vi "arduino_only.vi"() -> ()   [LabVIEW 2012]
panel:
  in  "Tab Control":T1(tab)
  in  "VISA resource name":refnum<visa-resource-name>="COM3"
  in  "Slow Control On":bool
  in  "Write Enable":bool
  in  "File Path":path=path "D:/Users/reuterc/Desktop"
  out "directory exists - please wait":u8(slide)
  out "directory ok":bool
  in  "General Cluster":cluster{"Location":i16} {"Location" items=["Purdue", "NIKHEF", "Zurich", "???"]}
  in  "IP Address of NIST Time Server":string(combo)
  in  "HV Cluster":T2={"HV Power On/Off"=[], "Set Voltage"=[], "HV Tolerance (%)"=1.0}
  out "Slow Cluster":T3
  out "data":dbl[](array[numeric])
  in  "XOFF Character":u8=19 format="%.0x"
  in  "XON Character":u8=17 format="%.0x"
  in  "Arduino read rate (Hz)":dbl=1.0
  out "Arduino \nread failed":bool
  out "UTC format":bool=TRUE
  out "read buffer":string
  out "Temperature":dbl(graph)
  out "Pressure":dbl(graph)
  out "total magnetic field":dbl(graph)
  out "magnetic field z coordinate":dbl(graph)
  out "magnetic field y coordinate":dbl(graph)
  out "magnetic field x coordinate":dbl(graph)
  out "humidity":dbl(graph)
  out "Slow XML":string
  out "NIST Time":u64
  out "Slow time":u64
  in  "Minutes to wait":u32=5 min=3
  out "NIST Time Failed to Read":bool
  out "created path":path
  out "File name":string
  out "Stopped":bool
  in  "stop 2":bool
  in  "stop":bool
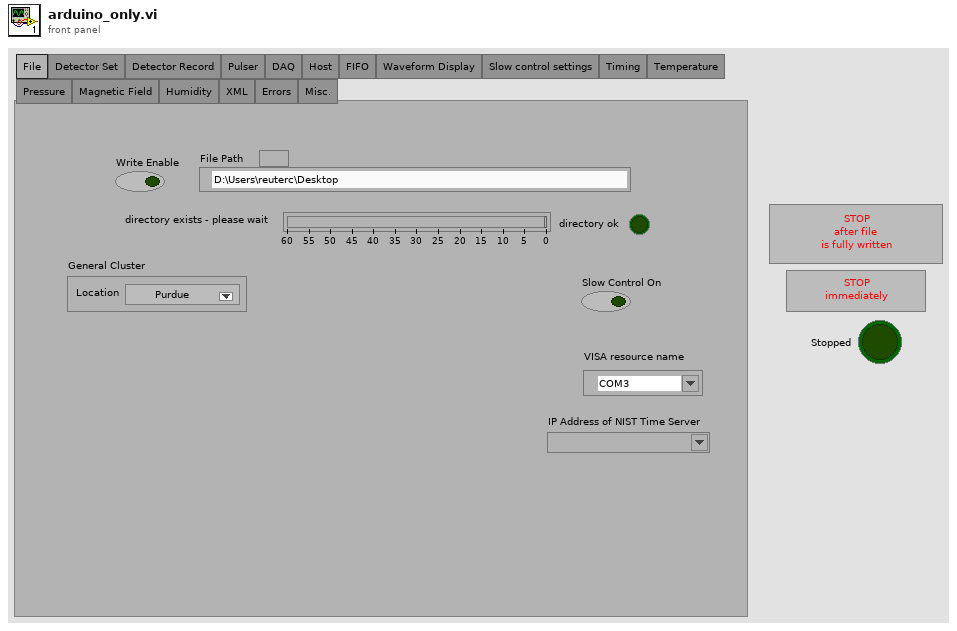
[diagram p1: front panel]
types:
  T1 = enum32{"File", "Detector Set", "Detector Record", "Pulser", "DAQ", "Host", "FIFO", "Waveform Display", "Slow control settings", "Timing", "Temperature", "Pressure", "Magnetic Field", "Humidity", "XML", "Errors", "Misc."}
  T2 = cluster{"HV Power On/Off":bool[], "Set Voltage":string[], "HV Tolerance (%)":dbl}
  T3 = cluster{"Arduino Parameters":dbl, "Total Number of Slow Parameters":i32, "UTC format?":bool, "Sensor Upper bounds":i32[], "Sensor Lower bounds":i32[], "Descriptions":string[], "datanames":string[]}
  T4 = enum16{"open", "replace", "create", "open or create", "replace or create", "replace or create with confirmation"}
  T5 = enum16{"big-endian, network order", "native, host order", "little-endian"}
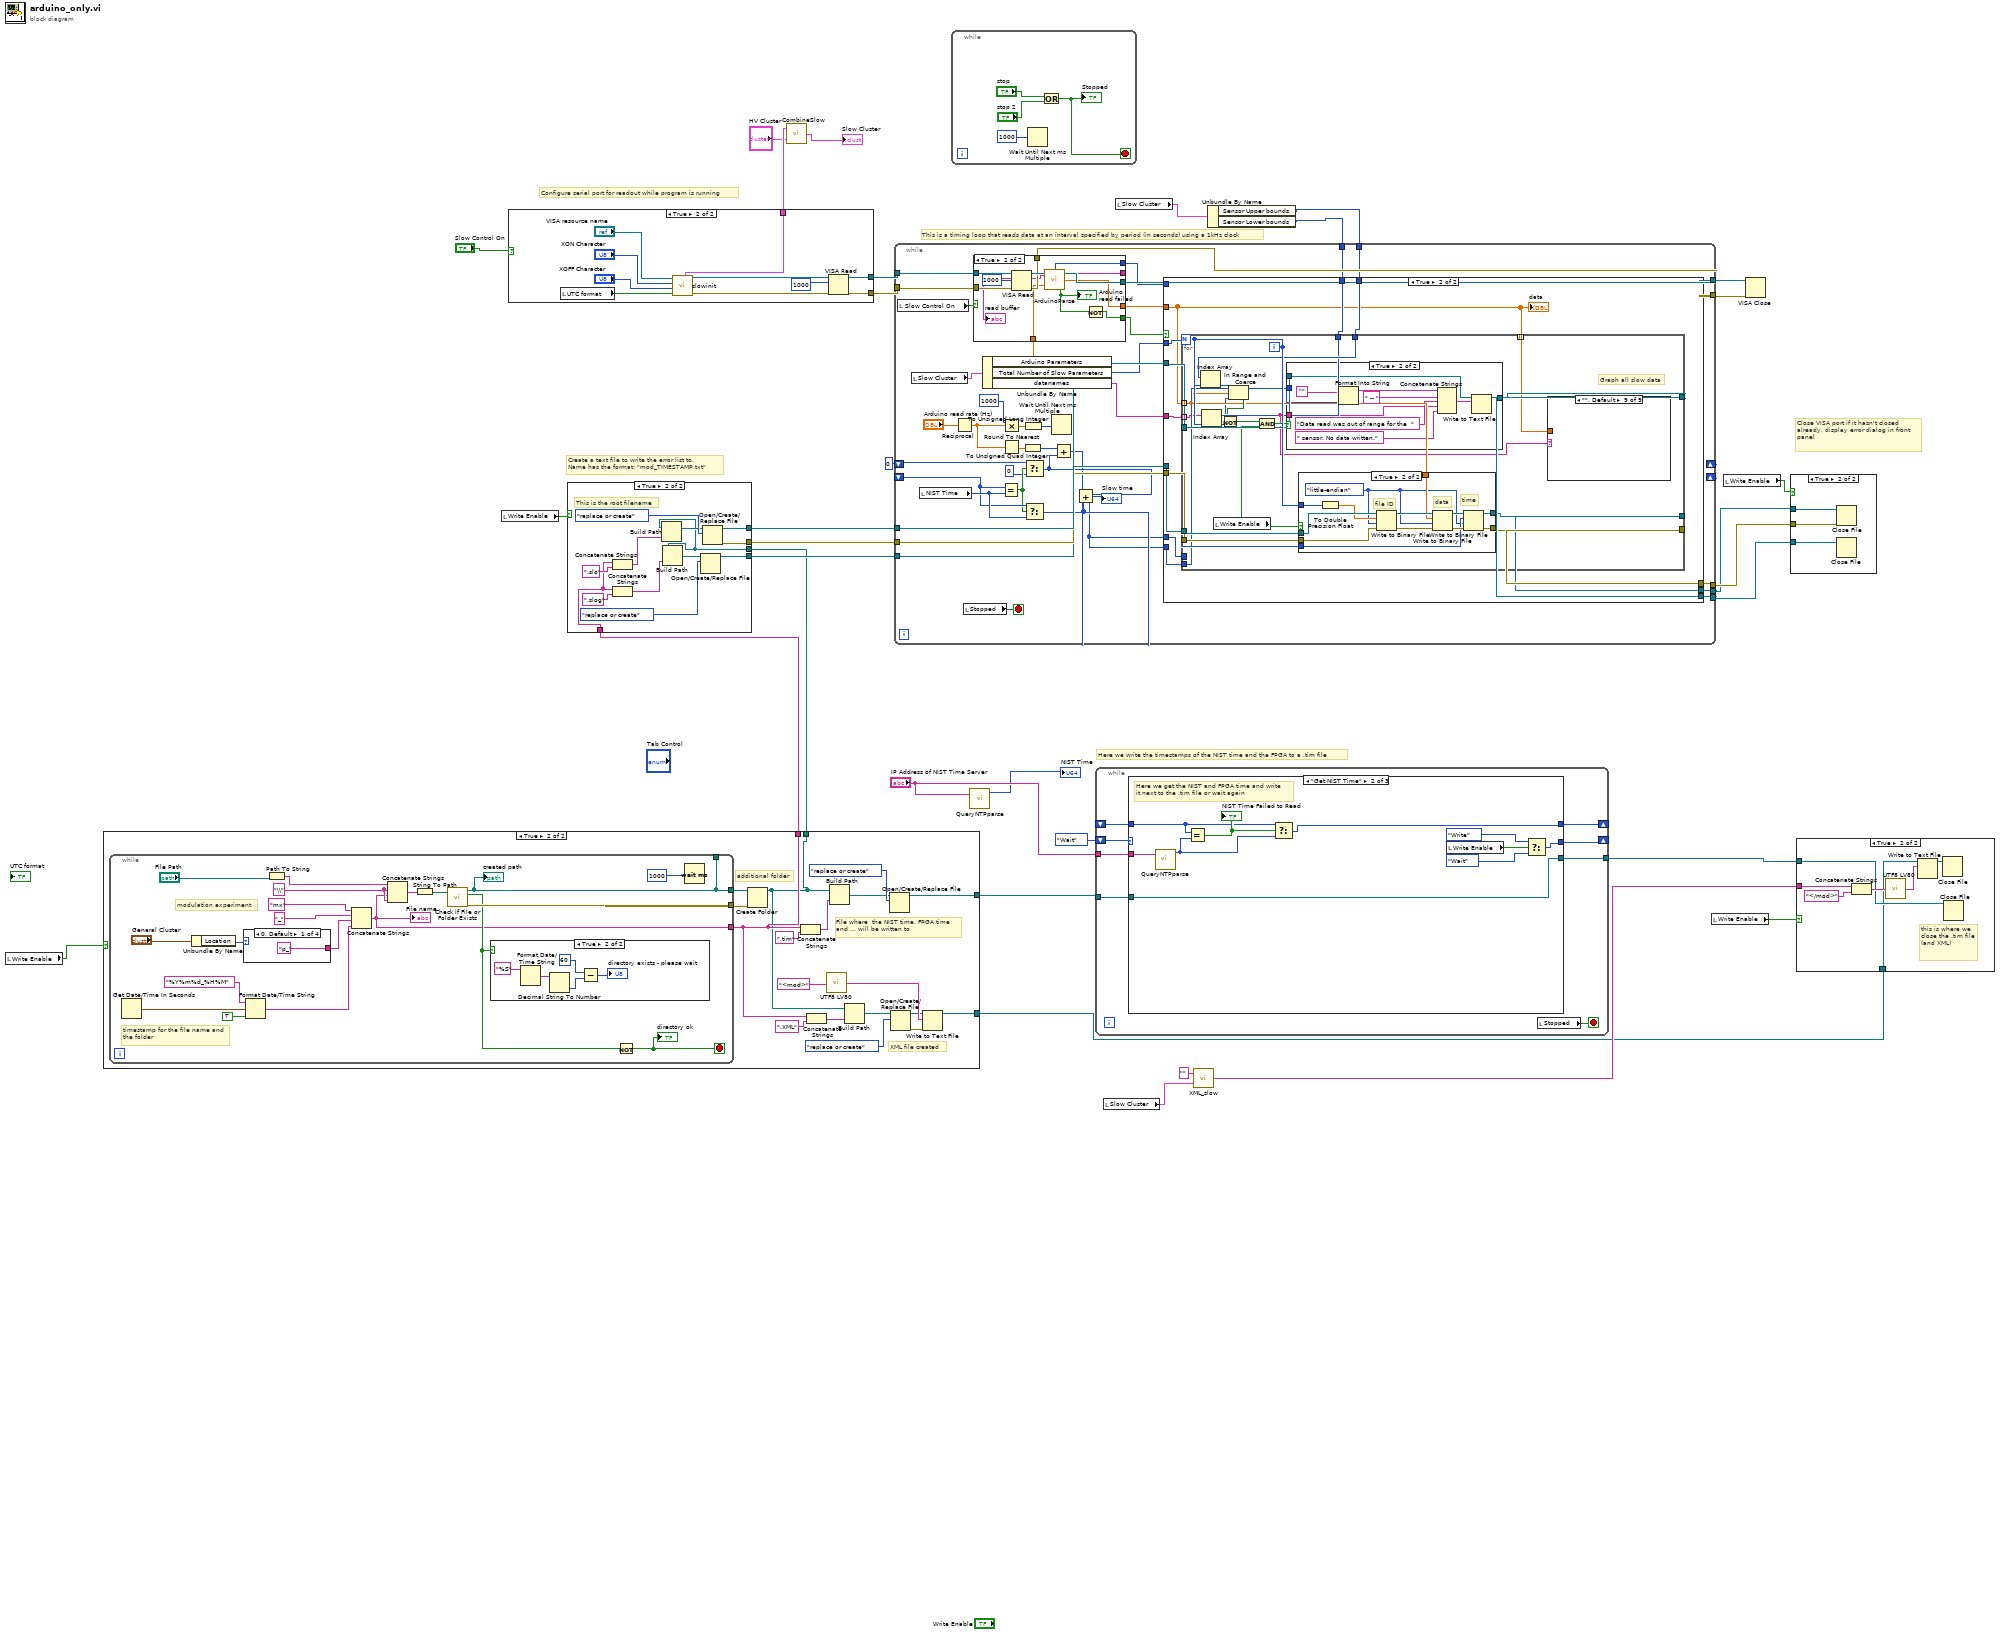
[diagram p0: block diagram]
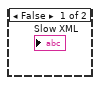
[diagram p3: hidden frame]
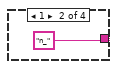
[diagram p4: hidden frame]
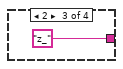
[diagram p5: hidden frame]
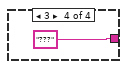
[diagram p6: hidden frame]
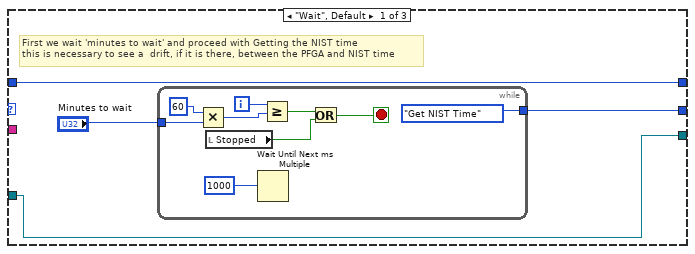
[diagram p8: hidden frame]
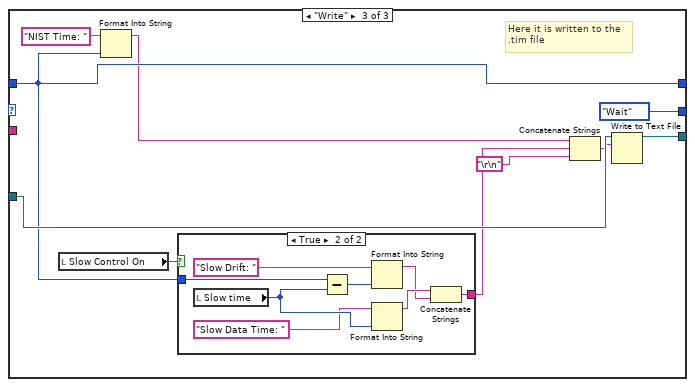
[diagram p9: hidden frame]
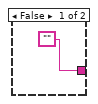
[diagram p10: hidden frame]
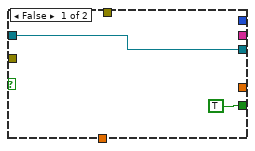
[diagram p12: hidden frame]
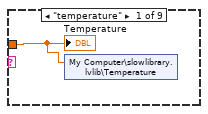
[diagram p14: hidden frame]
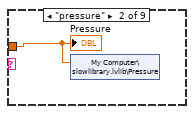
[diagram p15: hidden frame]
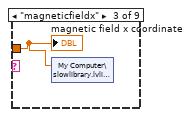
[diagram p16: hidden frame]
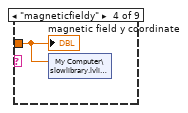
[diagram p17: hidden frame]
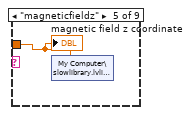
[diagram p18: hidden frame]
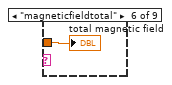
[diagram p19: hidden frame]
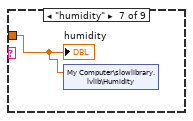
[diagram p20: hidden frame]
diagram:
  # "Here we write the timestamps of the NIST time and the FPGA to a .tim file"
  # "Create a text file to write the error list to.  \nName has the format: \"mod_TIMESTAMP.txt\""
  # "This is a timing loop that reads data at an interval specified by period (in seconds) using a 1kHz clock"
  # "Configure serial port for readout while program is running"
  # "Close VISA port if it hasn't closed already, display error dialog in front panel"
  n1 = local read "Write Enable"() -> (w4:bool)
  n2 = case shown="True" w4 {
    tunnel: [_ w38] -> w11
    tunnel: [_ w37] -> w5
    tunnel: [_ w36] -> w3
    tunnel: [_ w34] -> w1
    frame False {
    }
    frame True {
      # "XML file created"
      # "File where  the NIST time, FPGA time\nand ... will be written to"
      # "additional folder"
      n3 = while {
        tunnel: [w64] -> w47
        tunnel: [w56] -> w48
        tunnel: [w56] -> _
        tunnel: [w55] -> w36
        stop <- w61 stop-if-true
        w57 = "\\" ("string")
        # "modulation experiment"
        # "timestamp for the file name and the folder"
        n4 = Get Date/Time In Seconds() -> (seconds since 1Jan1904=w68:timestamp)
        n5 = Unbundle By Name("General Cluster") -> ("Location"=w53:i16)
        n6 = case shown="0, Default" w53 {
          tunnel: ["p_" ("string") "n_" ("string") "z_" ("string") "???"] -> w54
          frame 0, Default {
          }
          frame 1 {
          }
          frame 2 {
          }
          frame 3 {
          }
        }
        n7 = Format Date/Time String(time format string (%c)="%Y%m%d_%H%M", seconds (now)=w68, UTC format=TRUE) -> (date/time string=w58:string)
        n8 = Path To String(path="File Path") -> (string=w70:string)
        n9 = Concatenate Strings("mx" ("string"), "_" ("string"), w54, w58) -> (w55:string)
        "File name" <- w55
        n10 = Concatenate Strings(w70, w57, w55, w57) -> (w71:string)
        n11 = String To Path(string=w71) -> (path=w65:path)
        n12 = call <vilib>:"Check if File or Folder Exists.vi"("path"=w65) -> ("error out"=w64:errorcluster, "file or folder exists?"=w63:bool, "dup path"=w56:path)  [unwired: 8 in]
        "created path" <- w56
        n13 = case shown="True" w63 {
          frame False {
          }
          frame True {
            n14 = Format Date/Time String(time format string (%c)="%S") -> (date/time string=w79:string)  [unwired: 2 in]
            n15 = Decimal String To Number(string=w79) -> (number=w77:i32)  [unwired: 2 in, 1 out]
            n16 = Subtract(x=60, y=w77) -> (x-y=→"directory exists - please wait":i32)
          }
        }
        n17 = Not(x=w63) -> (.not. x?=w61:bool)
        "directory ok" <- w61
        n18 = Wait (ms)(milliseconds to wait=1000) -> ()  [unwired: 1 out]
      }
      n19 = Create Folder(path (use dialog)=w48, error in=w47) -> (created path=w34:path)  [unwired: 1 in, 2 out]
      n20 = Concatenate Strings(w36, ".tim" ("string")) -> (w49:string)
      n21 = Concatenate Strings(w36, ".XML" ("substring (\"\")")) -> (w43:string)
      n22 = call "UTF8 LV80.vi"("text"="<mod>") -> ("utf-8 text out"=w46:string)
      n23 = Build Path(base path=w34, name or relative path=w49) -> (appended path=w35:path)
      n24 = Build Path(base path=w34, name or relative path=w43) -> (appended path=w42:path)
      n25 = Open/Create/Replace File(file path (use dialog)=w35, operation (0:open)=T4."replace or create") -> (refnum out=w38:refnum<file>)  [unwired: 4 in, 2 out]
      n26 = Open/Create/Replace File(file path (use dialog)=w42, operation (0:open)=T4."replace or create") -> (refnum out=w45:refnum<file>, error out=w44:errorcluster)  [unwired: 4 in, 1 out]
      n27 = Write to Text File(file (use dialog)=w45, text=w46, error in=w44) -> (refnum out=w37:refnum<file>)  [unwired: 1 in, 2 out]
    }
  }
  n28 = local read "Write Enable"() -> (w32:bool)
  n29 = case shown="True" "Slow Control On" {
    tunnel: [_ w90] -> w24
    tunnel: [_ w89] -> w23
    tunnel: [_ w81] -> w16
    frame False {
    }
    frame True {
      n30 = local read "UTC format"() -> (w84:bool)
      n31 = call "slowinit.vi"("UTC format"=w84, "XOFF Character"="XOFF Character", "XON Character"="XON Character", "VISA resource name"="VISA resource name") -> ("error IO"=w82:errorcluster, "VISA resource name out"=w83:refnum<visa-resource-name>, "Slow Cluster"=w81:T3)  [unwired: 5 in]
      n32 = VISA Read(VISA resource name=w83, byte count=u32 1000, error in (no error)=w82) -> (VISA resource name out=w90:refnum<visa-resource-name>, error out=w89:errorcluster)  [unwired: 2 out]
    }
  }
  n33 = case shown="True" w32 {
    tunnel: [_ w101] -> w29
    tunnel: [_ w98] -> w27
    tunnel: [_ w93] -> w22
    tunnel: w3 -> [_ w92]
    tunnel: w1 -> [_ w91]
    frame False {
    }
    frame True {
      # "This is the root filename"
      n34 = Concatenate Strings(w92, ".slo") -> (w99:string)
      n35 = Concatenate Strings(w92, ".slog") -> (w94:string)
      n36 = Build Path(base path=w91, name or relative path=w99) -> (appended path=w100:path)
      n37 = Build Path(base path=w91, name or relative path=w94) -> (appended path=w95:path)
      n38 = Open/Create/Replace File(file path (use dialog)=w95, operation (0:open)=T4."replace or create") -> (refnum out=w93:refnum<file>)  [unwired: 4 in, 2 out]
      n39 = Open/Create/Replace File(file path (use dialog)=w100, operation (0:open)=T4."replace or create") -> (refnum out=w101:refnum<file>, error out=w98:errorcluster)  [unwired: 4 in, 1 out]
    }
  }
  n40 = call "CombineSlow.vi"("HV Cluster"="HV Cluster", "Slow Cluster"=w16) -> ("Slow Cluster 2"=→"Slow Cluster":T3)
  n41 = while {
    stop <- w104 stop-if-true
    n42 = Wait Until Next ms Multiple(millisecond multiple=u32 1000 ("y")) -> ()  [unwired: 1 out]
    n43 = Or(x="stop", y="stop 2") -> (x .or. y?=w104:bool)
    "Stopped" <- w104
  }
  n44 = call "QueryNTPparse.vi"("IP Address of NIST Server"="IP Address of NIST Time Server") -> ("NTP Time"=→"NIST Time":u64)  [unwired: 1 in, 2 out]
  n45 = while {
    shift-right: [w114] -> _
    shift-left: enum16{"Wait", "Get NIST Time", "Write"}."Wait" -> [w115]
    shift-right: [w113] -> _
    shift-left: _ -> [w112]
    tunnel: w11 -> [w111]
    tunnel: [w110] -> w9
    tunnel: "IP Address of NIST Time Server" -> [w109]
    stop <- w108 stop-if-true
    n46 = case shown="\"Get NIST Time\"" w115 {
      tunnel: [w119 w130 enum16{"Wait", "Get NIST Time", "Write"}."Wait"] -> w114
      tunnel: [w118 w138 w143] -> w113
      tunnel: w112 -> [w118 w135 w143]
      tunnel: w111 -> [w117 w134 w147]
      tunnel: [w117 w134 w146] -> w110
      tunnel: w109 -> [_ w129 _]
      frame "Wait", Default {
        # "First we wait 'minutes to wait' and proceed with Getting the NIST time\nthis is necessary to see a  drift, if it is there, between the PFGA and NIST time"
        n47 = while {
          tunnel: [enum16{"Wait", "Get NIST Time", "Write"}."Get NIST Time"] -> w119
          tunnel: "Minutes to wait" -> [w122]
          i -> [w124]
          stop <- w125 stop-if-true
          n48 = Multiply(x=60, y=w122) -> (x*y=w121:u32)
          n49 = local read "Stopped"() -> (w120:bool)
          n50 = Wait Until Next ms Multiple(millisecond multiple=u32 1000 ("y")) -> ()  [unwired: 1 out]
          n51 = Greater Or Equal?(x=w124, y=w121) -> (x >= y?=w126:bool)
          n52 = Or(x=w126, y=w120) -> (x .or. y?=w125:bool)
        }
      }
      frame "Get NIST Time" {
        # "Here we get the NIST and FPGA time and write\nit next to the .tim file or wait again"
        n53 = call "QueryNTPparse.vi"("IP Address of NIST Server"=w129) -> ("NTP Time"=w137:u64)  [unwired: 1 in, 2 out]
        n54 = Equal?(x=w135, y=w137) -> (x = y?=w136:bool)
        "NIST Time Failed to Read" <- w136
        n55 = Select(t=w135, s=w136, f=w137) -> (s? t:f=w138:u64)
        n56 = local read "Write Enable"() -> (w133:bool)
        n57 = Select(t=enum16{"Wait", "Get NIST Time", "Write"}."Write", s=w133, f=enum16{"Wait", "Get NIST Time", "Write"}."Wait") -> (s? t:f=w130:enum16{"Wait", "Get NIST Time", "Write"})
      }
      frame "Write" {
        # "Here it is written to the \n.tim file"
        n58 = local read "Slow Control On"() -> (w140:bool)
        n59 = Format Into String(initial string="NIST Time: ", w143) -> (resulting string=w139:string)  [unwired: 2 in, 1 out]
        n60 = case shown="True" w140 {
          tunnel: w143 -> [_ w154]
          tunnel: ["" w150] -> w142
          frame False {
          }
          frame True {
            n61 = local read "Slow time"() -> (w157:u64)
            n62 = Subtract(x=w154, y=w157) -> (x-y=w153:u64)
            n63 = Format Into String(initial string="Slow Drift: ", w153) -> (resulting string=w151:string)  [unwired: 2 in, 1 out]
            n64 = Format Into String(initial string="Slow Data Time: ", w157) -> (resulting string=w152:string)  [unwired: 2 in, 1 out]
            n65 = Concatenate Strings(w152, w151) -> (w150:string)
          }
        }
        n66 = Concatenate Strings(w139, w142, "\r\n") -> (w145:string)
        n67 = Write to Text File(file (use dialog)=w147, text=w145) -> (refnum out=w146:refnum<file>)  [unwired: 2 in, 2 out]
      }
    }
    n68 = local read "Stopped"() -> (w108:bool)
  }
  n69 = local read "Slow Cluster"() -> (w7:T3)
  n70 = local read "Slow Cluster"() -> (w20:T3)
  n71 = call "XML_slow.vi"("Slow Cluster"=w7, "Input String"="") -> ("Output String"=w6:string)
  n72 = Unbundle By Name(w20) -> ("Sensor Upper bounds"=w19:i32[], "Sensor Lower bounds"=w18:i32[])
  n73 = while {
    tunnel: w24 -> [w194]
    tunnel: w23 -> [w193]
    tunnel: [w192] -> w31
    tunnel: [w191] -> w30
    shift-right: [w184] -> _
    shift-left: _ -> [w188]
    shift-right: [w173] -> _
    shift-left: 0 -> [w186]
    tunnel: w27 -> [w182]
    tunnel: [w181] -> w26
    tunnel: w29 -> [w190]
    tunnel: [w180] -> w25
    tunnel: w22 -> [w179]
    tunnel: [w177] -> w21
    tunnel: w19 -> [w165]
    tunnel: w18 -> [w164]
    stop <- w183 stop-if-true
    n74 = local read "Slow Control On"() -> (w161:bool)
    n75 = local read "Slow Cluster"() -> (w167:T3)
    n76 = local read "NIST Time"() -> (w189:u64)
    n77 = Reciprocal(x="Arduino read rate (Hz)") -> (1/x=w170:dbl)
    n78 = local read "Stopped"() -> (w183:bool)
    n79 = Unbundle By Name(w167) -> ("Arduino Parameters"=w162:dbl, "Total Number of Slow Parameters"=w163:i32, "datanames"=w159:string[])
    n80 = case shown="True" w161 {
      tunnel: w194 -> [w195 w207]
      tunnel: w193 -> [_ w206]
      tunnel: [w195 w205] -> w192
      tunnel: [_ w204] -> w191
      tunnel: [_ w202] -> w166
      tunnel: [_ w201] -> _
      tunnel: [TRUE w197] -> w160
      tunnel: [_ w199] -> w158
      tunnel: w162 -> [_ w198]
      frame False {
      }
      frame True {
        n81 = VISA Read(VISA resource name=w207, byte count=u32 1000, error in (no error)=w206) -> (VISA resource name out=w205:refnum<visa-resource-name>, read buffer=w203:string, error out=w204:errorcluster)  [unwired: 1 out]
        "read buffer" <- w203
        n82 = call "ArduinoParse.vi"("read buffer"=w203, "Expected Arduino Parameters"=w198) -> ("Number Arduino Parameters"=w202:i32, "Arduino Data Names"=w201:string[], "Arduino Data"=w199:dbl[], "Arduino Read Failed?"=w200:bool)
        "Arduino \nread failed" <- w200
        n83 = Not(x=w200) -> (.not. x?=w197:bool)
      }
    }
    n84 = Equal?(x=w188, y=w189) -> (x = y?=w187:bool)
    n85 = Multiply(x=u32 1000 ("millisecond multiple"), y=w170) -> (x*y=w172:dbl)
    n86 = Round To Nearest(number=w170) -> (nearest integer value=w169:dbl)
    n87 = To Unsigned Quad Integer(1:w169) -> (0:w168:u64)
    n88 = To Unsigned Long Integer(number=w172) -> (unsigned 32bit integer=w171:u32)
    n89 = Select(t=w186, s=w187, f=0) -> (s? t:f=w174:u64)
    n90 = Select(t=w188, s=w187, f=w189) -> (s? t:f=w184:u64)
    n91 = Wait Until Next ms Multiple(millisecond multiple=w171) -> ()  [unwired: 1 out]
    n92 = Add(x=w168, y=w174) -> (x+y=w173:u64)
    n93 = Add(x=w174, y=w184) -> (x+y=w178:u64)
    "Slow time" <- w178
    n94 = case shown="True" w160 {
      tunnel: w190 -> [w210 w224]
      tunnel: w178 -> [_ w223]
      tunnel: w182 -> [w211 w222]
      tunnel: [w211 w221] -> w181
      tunnel: [w210 w220] -> w180
      tunnel: w179 -> [w209 w219]
      tunnel: w178 -> [_ w218]
      tunnel: [w209 w217] -> w177
      tunnel: w166 -> [_ _]
      tunnel: w158 -> [_ w212]
      tunnel: w159 -> [_ w216]
      tunnel: w165 -> [_ w215]
      tunnel: w164 -> [_ w214]
      tunnel: w163 -> [_ w213]
      frame False {
      }
      frame True {
        n95 = for {
          N: w213 -> [_]
          tunnel: w224 -> [w244]
          tunnel: [w243] -> w220
          tunnel: w223 -> [w242]
          tunnel: w222 -> [w241]
          tunnel: [w240] -> w221
          tunnel: w219 -> [w238]
          tunnel: w218 -> [w237]
          tunnel: [w236] -> w217
          tunnel: w215 -> [w233]
          tunnel: w214 -> [w232]
          tunnel: w212 -> [w230] mode=indexing
          tunnel: w216 -> [w226] mode=indexing
          tunnel: w212 -> [w225] mode=indexing
          i -> [w239]
          # "Graph all slow data"
          n96 = Index Array(array=w233, index=w239) -> (element=w229:i32)
          n97 = Index Array(array=w232, index=w239) -> (element=w228:i32)
          n98 = local read "Write Enable"() -> (w227:bool)
          n99 = In Range and Coerce(upper limit=w229, x=w230, lower limit=w228) -> (In Range?=w231:bool)  [unwired: 1 out]
          n100 = Not(x=w231) -> (.not. x?=w235:bool)
          n101 = And(x=w235, y=w227) -> (x .and. y?=w234:bool)
          n102 = case shown="True" w234 {
            tunnel: w238 -> [w252 w260]
            tunnel: w237 -> [_ w258]
            tunnel: [w252 w256] -> w236
            tunnel: w226 -> [_ w253]
            frame False {
            }
            frame True {
              n103 = Format Into String(initial string="", w258) -> (resulting string=w257:string)  [unwired: 2 in, 1 out]
              n104 = Concatenate Strings(w257, " -- " ("format string"), "Data read was out of range for the  " ("format string"), w253, " sensor. No data written." ("format string")) -> (w254:string)
              n105 = Write to Text File(file (use dialog)=w260, text=w254) -> (refnum out=w256:refnum<file>)  [unwired: 2 in, 2 out]
            }
          }
          n106 = case shown="True" w227 {
            tunnel: [w264 w271] -> w243
            tunnel: w244 -> [w264 w274]
            tunnel: w239 -> [_ w275]
            tunnel: w242 -> [_ w268]
            tunnel: w241 -> [w263 w277]
            tunnel: [w263 w269] -> w240
            tunnel: w230 -> [_ w267]
            frame False {
            }
            frame True {
              w265 = T5."little-endian" ("byte order (0:big-endian, network order)")
              # "time"
              # "data"
              # "file ID"
              n107 = To Double Precision Float(number=w275) -> (double precision float=w266:dbl)
              n108 = Write to Binary File(file (use dialog)=w274, data=w266, error in=w277, 9:w265) -> (refnum out=w273:refnum<file>, error out=w276:errorcluster)  [unwired: 2 in, 1 out]
              n109 = Write to Binary File(file (use dialog)=w273, data=w267, error in=w276, 9:w265) -> (refnum out=w272:refnum<file>, error out=w270:errorcluster)  [unwired: 2 in, 1 out]
              n110 = Write to Binary File(file (use dialog)=w272, data=w268, error in=w270, 9:w265) -> (refnum out=w271:refnum<file>, error out=w269:errorcluster)  [unwired: 2 in, 1 out]
            }
          }
          n111 = case shown="\"\", Default" w226 {
            tunnel: w225 -> [w245 w246 w247 w248 w249 w250 w251 _ _]
            frame "temperature" {
              n112 = shared-variable "My Computer\\slowlibrary.lvlib\\Temperature"(w245) -> ()  [unwired: 1 in, 1 out]
              "Temperature" <- w245
            }
            frame "pressure" {
              n113 = shared-variable "My Computer\\slowlibrary.lvlib\\Pressure"(w246) -> ()  [unwired: 1 in, 1 out]
              "Pressure" <- w246
            }
            frame "magneticfieldx" {
              n114 = shared-variable "My Computer\\slowlibrary.lvlib\\B_x"(w247) -> ()  [unwired: 1 in, 1 out]
              "magnetic field x coordinate" <- w247
            }
            frame "magneticfieldy" {
              n115 = shared-variable "My Computer\\slowlibrary.lvlib\\B_y"(w248) -> ()  [unwired: 1 in, 1 out]
              "magnetic field y coordinate" <- w248
            }
            frame "magneticfieldz" {
              n116 = shared-variable "My Computer\\slowlibrary.lvlib\\B_z"(w249) -> ()  [unwired: 1 in, 1 out]
              "magnetic field z coordinate" <- w249
            }
            frame "magneticfieldtotal" {
              "total magnetic field" <- w250
            }
            frame "humidity" {
              n117 = shared-variable "My Computer\\slowlibrary.lvlib\\Humidity"(w251) -> ()  [unwired: 1 in, 1 out]
              "humidity" <- w251
            }
            frame "seconds" {
            }
            frame "", Default {
            }
          }
        }
        "data" <- w212
      }
    }
  }
  n118 = local read "Write Enable"() -> (w10:bool)
  n119 = local read "Write Enable"() -> (w33:bool)
  n120 = VISA Close(VISA resource name=w31, error in (no error)=w30) -> ()  [unwired: 1 out]
  n121 = case shown="True" w33 {
    tunnel: w25 -> [_ w280]
    tunnel: w26 -> [_ w279]
    tunnel: w21 -> [_ w278]
    frame False {
    }
    frame True {
      n122 = Close File(refnum=w278) -> ()  [unwired: 1 in, 2 out]
      n123 = Close File(refnum=w280, error in=w279) -> ()  [unwired: 2 out]
    }
  }
  n124 = case shown="True" w10 {
    tunnel: w9 -> [_ w282]
    tunnel: w6 -> [_ w283]
    tunnel: w5 -> [_ w281]
    frame False {
    }
    frame True {
      # "this is where we close the .tim file (and XML)"
      n125 = Concatenate Strings(w283, "</mod>" ("string")) -> (w284:string)
      n126 = call "UTF8 LV80.vi"("text"=w284) -> ("utf-8 text out"=w287:string)
      n127 = Write to Text File(file (use dialog)=w281, text=w287) -> (refnum out=w286:refnum<file>)  [unwired: 2 in, 2 out]
      n128 = Close File(refnum=w286) -> ()  [unwired: 1 in, 2 out]
      n129 = Close File(refnum=w282) -> ()  [unwired: 1 in, 2 out]
    }
  }
